vi "J1939LoopBackTest.vi"() -> ()   [LabVIEW 2013, in "J1939 tests.lvlib"]
uses:
  J1939 tests.lvlib
  <vilib>/xnet/xnet.llb/XNET Create Session (Signal Output Single-point).vi
  module/execution/J1939 Claim With Address.vi
  <vilib>/xnet/xnet.llb/XNET Create Session (Signal Input Single-point).vi
  <vilib>/xnet/xnet.llb/XNET Write (Signal Single-point).vi
  <vilib>/xnet/xnet.llb/XNET Read (Signal Single-point).vi
  module/execution/J1939 runtime.lvclass
  <resource>/objmgr/xnet.rc
panel:
  out "Database":refnum<k21>
  in  "Node Address 2":u8
  in  "stop 2":bool
  in  "Write":bool
  in  "Signal Single Point Data 2":dbl[](array[knob])=[0.0, 0.0] caption="data" scale=0.0..50.0
  in  "Select Interface 2":refnum<k21>="CAN1"
  in  "Select Signal List from database 2":refnum<k21>[](array[refnum])=["J1939_LargeSignal1\nNIXNET_example.J1939_Over_CAN", "J1939_LargeSignal2\nNIXNET_example.J1939_Over_CAN"]
  in  "Node Address":u8=1
  in  "stop":bool
  out "Signal Single Point Data":dbl[](array[knob]) caption="data" scale=0.0..50.0
  in  "Update":bool
  in  "Select Interface":refnum<k21>="CAN2"
  out "Select Signal List from database":refnum<k21>[](array[refnum])=["J1939_LargeSignal1\nNIXNET_example.J1939_Over_CAN", "J1939_LargeSignal2\nNIXNET_example.J1939_Over_CAN"]
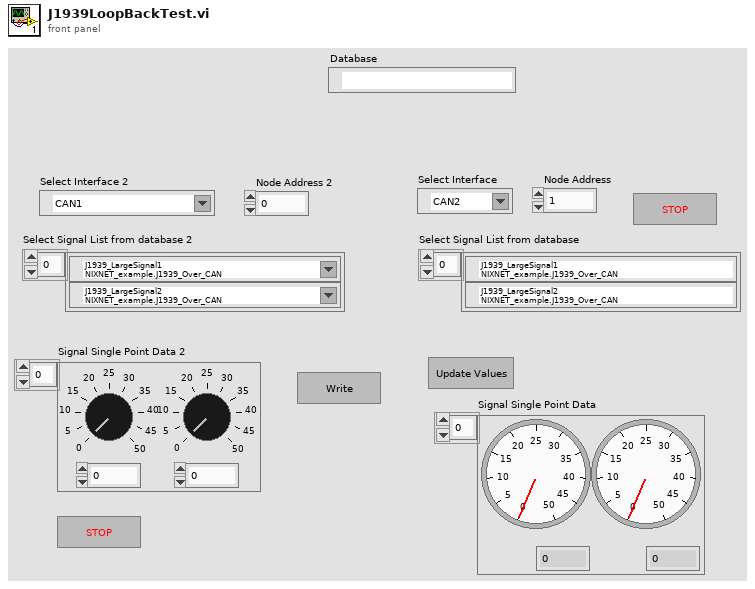
[diagram p1: front panel]
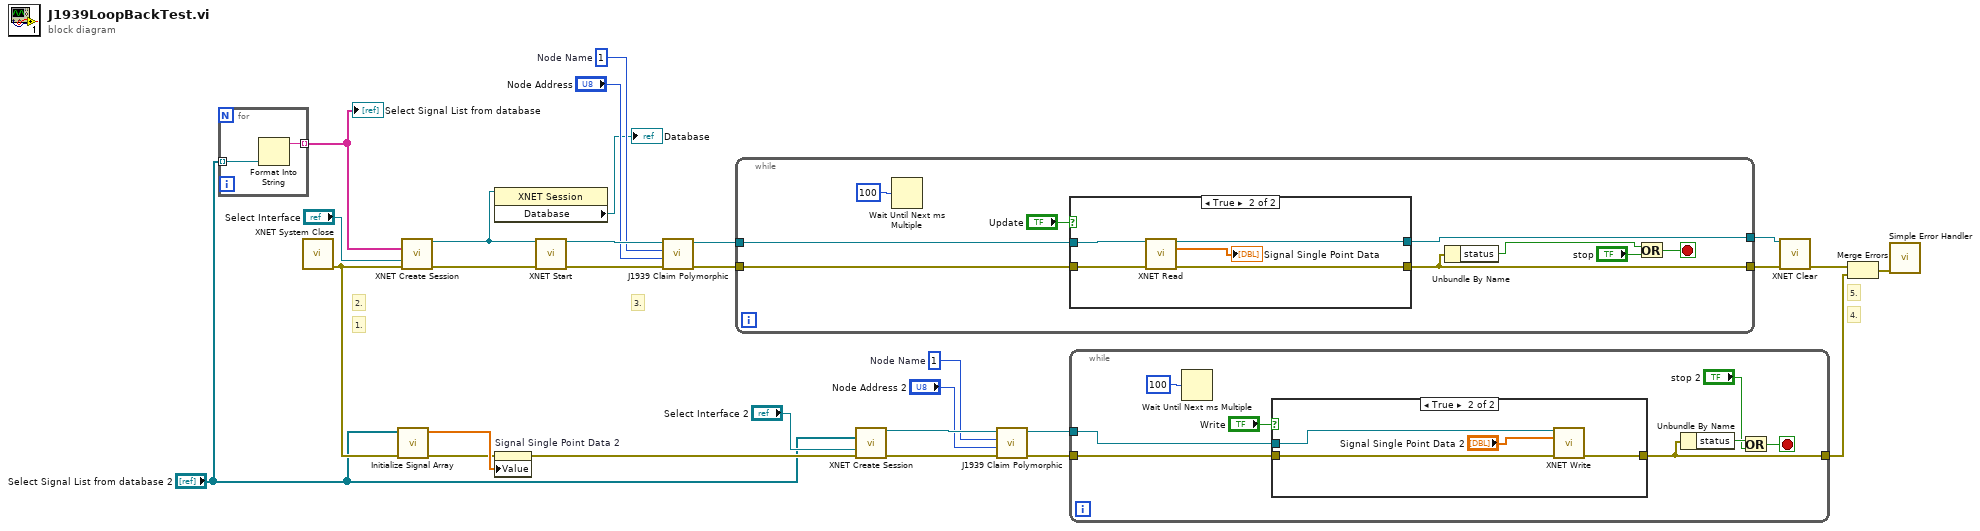
[diagram p0: block diagram]
diagram:
  w8 = u64 1  # Node Name
  w19 = u64 1  # Node Name
  # "3."
  # "5."
  # "2."
  # "4."
  # "1."
  n1 = for {
    tunnel: "Select Signal List from database 2" -> [w30] mode=indexing
    tunnel: [w29] -> w5 mode=indexing
    n2 = Format Into String(w30) -> (resulting string=w29:string)  [unwired: 3 in, 1 out]
  }
  "Select Signal List from database" <- w5
  n3 = call <vilib>:"XNET System Close.vi"() -> ("error out"=w7:errorcluster)  [unwired: 15 in]
  n4 = call "Initialize Signal Array.vi"("error out"=w7, "signal list"="Select Signal List from database 2") -> ("error out"=w15:errorcluster, "Array"=w16:dbl[])  [unwired: 6 out]
  n5 = call-poly <vilib>:"XNET Create Session.vi"("signal list"=w5, "interface"="Select Interface", "error in (no error)"=w7) -> ("session out"=w4:refnum<k21>, "error out"=w27:errorcluster)  [unwired: 11 out]
  n6 = property class="XNET Session"(reference=w4) -> ("Database"=→"Database":refnum<k21>)  [unwired: 1 in, 2 out]
  n7 = property on="Signal Single Point Data 2" class="Arr (strict)"(error in=w15, "Value"=w16) -> (error out=w14:errorcluster)  [unwired: 1 in, 1 out]
  n8 = call <vilib>:"XNET Start.vi"("session in"=w4, "error in (no error)"=w27) -> ("session out"=w23:refnum<k21>, "error out"=w22:errorcluster)  [unwired: 12 in]
  n9 = call-poly "J1939 Claim Polymorphic.vi"("error in (no error)"=w22, "SAE J1939:Node Address"="Node Address", "SAE J1939:Node Name"=w19, "XNET Session"=w23) -> ("error out"=w21:errorcluster, "XNET Session Out"=w20:refnum<k21>)  [unwired: 5 in, 1 out]
  n10 = while {
    tunnel: [w39] -> w26
    tunnel: w20 -> [w35]
    tunnel: w21 -> [w34]
    tunnel: [w31] -> w24
    stop <- w36 stop-if-true
    n11 = Wait Until Next ms Multiple(millisecond multiple=u32 100 ("milliseconds to wait")) -> ()  [unwired: 1 out]
    n12 = case shown="True" "Update" {
      tunnel: [w41 w46] -> w39
      tunnel: w35 -> [w40 w44]
      tunnel: w34 -> [w41 w43]
      tunnel: [w40 w42] -> w31
      frame False {
      }
      frame True {
        n13 = call-poly <vilib>:"XNET Read.vi"("session in"=w44, "error in (no error)"=w43) -> ("session out"=w42:refnum<k21>, "data"=→"Signal Single Point Data":dbl[], "error out"=w46:errorcluster)  [unwired: 11 out]
      }
    }
    n14 = Unbundle By Name(w39) -> ("status"=w38:bool)
    n15 = Or(x=w38, y="stop") -> (x .or. y?=w36:bool)
  }
  n16 = call-poly <vilib>:"XNET Create Session.vi"("signal list"="Select Signal List from database 2", "interface"="Select Interface 2", "error in (no error)"=w14) -> ("session out"=w13:refnum<k21>, "error out"=w12:errorcluster)  [unwired: 11 out]
  n17 = call-poly "J1939 Claim Polymorphic.vi"("error in (no error)"=w12, "SAE J1939:Node Address"="Node Address 2", "SAE J1939:Node Name"=w8, "XNET Session"=w13) -> ("error out"=w11:errorcluster, "XNET Session Out"=w10:refnum<k21>)  [unwired: 5 in, 1 out]
  n18 = while {
    tunnel: w10 -> [w52]
    tunnel: w11 -> [w51]
    tunnel: [w50] -> w1
    stop <- w53 stop-if-true
    n19 = Wait Until Next ms Multiple(millisecond multiple=u32 100 ("milliseconds to wait")) -> ()  [unwired: 1 out]
    n20 = case shown="True" "Write" {
      tunnel: w52 -> [_ w59]
      tunnel: w51 -> [w55 w58]
      tunnel: [w55 w57] -> w50
      frame False {
      }
      frame True {
        n21 = call-poly <vilib>:"XNET Write.vi"("session in"=w59, "data"="Signal Single Point Data 2", "error in (no error)"=w58) -> ("error out"=w57:errorcluster)  [unwired: 12 out]
      }
    }
    n22 = Unbundle By Name(w50) -> ("status"=w54:bool)
    n23 = Or(x=w54, y="stop 2") -> (x .or. y?=w53:bool)
  }
  n24 = call <vilib>:"XNET Clear.vi"("session in"=w24, "error in (no error)"=w26) -> ("error out"=w25:errorcluster)  [unwired: 13 in]
  n25 = Merge Errors(w25, w1) -> (w2:errorcluster)
  n26 = call <vilib>:"Simple Error Handler.vi"("error in (no error)"=w2) -> ()  [unwired: 1 in, 8 out]
